vi "Value Change.vi"(8 "error in (no error)":errorcluster, 9 "NewVal":i32[](array[numeric]), 10 "Debugger":refnum<class "Debug Process.lvclass">, 11 "List Box View Model In":refnum<class "List Box View Model.lvclass">) -> (0 "error out":errorcluster, 3 "List Box View Model Out":refnum<class "List Box View Model.lvclass">)   [LabVIEW 2020, in "List Box View Model.lvclass"]
uses:
  List Box View Model.lvclass
  Process/Debug Process.lvclass
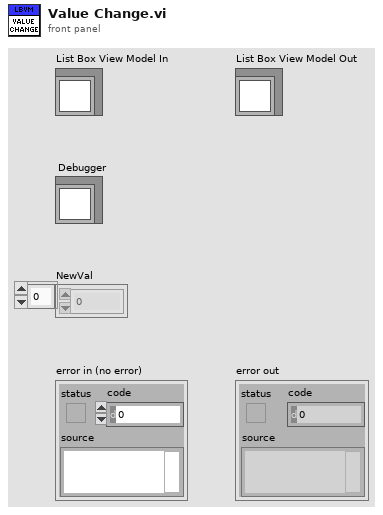
[diagram p1: front panel]
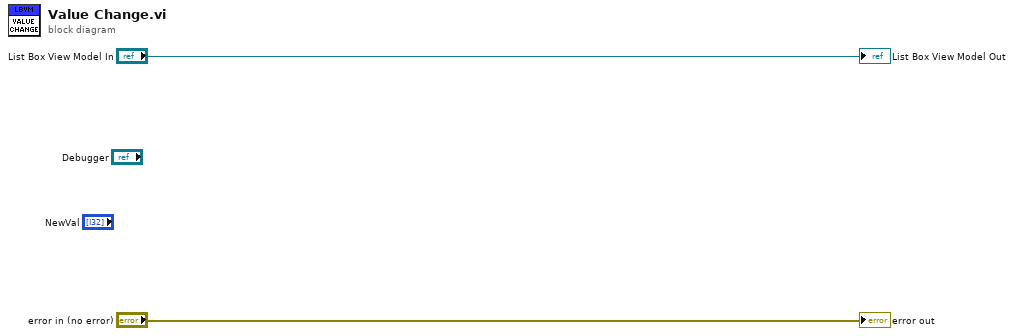
[diagram p0: block diagram]
diagram:
  "error out" <- "error in (no error)"
  "List Box View Model Out" <- "List Box View Model In"
